vi "enter-registration1.vi"(1 "OK":bool caption="ZATWIERDZ", 2 "registration":string caption="Wprowadz rejestracje", 3 "input array":string[](array[string])) -> (0 "output array":string[](array[string]))   [LabVIEW 2023]
doc: "Ten subVI przyjmuje tablice jako wejscie oraz w wolne miejsce w tej tablicy wpisuje numer rejestracji i zwraca tablice ze wpisana rejestracja."
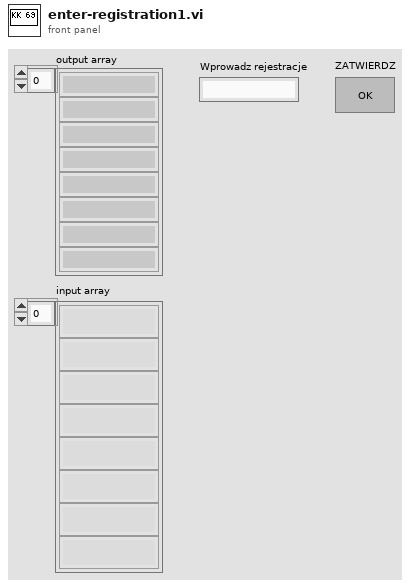
[diagram p1: front panel]
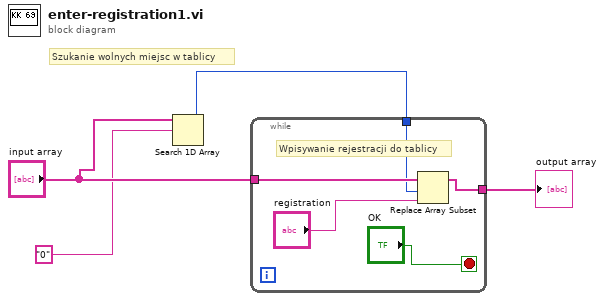
[diagram p0: block diagram]
diagram:
  # "Szukanie wolnych miejsc w tablicy"
  n1 = Search 1D Array(1D array="input array", element="0") -> (index of element=w4:i32)  [unwired: 1 in]
  n2 = while {
    tunnel: "input array" -> [w9]
    tunnel: w4 -> [w8]
    tunnel: [w7] -> w3
    stop <- "OK" stop-if-true
    # "Wpisywanie rejestracji do tablicy"
    n3 = Replace Array Subset(array=w9, new element="registration", index=w8) -> (w7:string[])
  }
  "output array" <- w3
